vi "Configure External Clock.vi"(0 "device session in":refnum<class "Device Session.lvclass">, 5 "external clock source":T1, 7 "external clock rate (Hz)":dbl=250000000.0 format="%#_6p", 11 "error in":errorcluster) -> (4 "device session out":refnum<class "Device Session.lvclass">, 6 "actual adc clock rate (Hz)":dbl=250000000.0 format="%#_6p", 15 "error out":errorcluster)   [LabVIEW 2021, in "Device Session.lvclass"]
doc: "Selects an external clock source and configures the external clock rate. When using an external clock, you must run the <B>Disable Data Clock</B> VI before disconnecting the external clock source.\n\n<B>Input Parameters</B>\n\n<B>device session in</B> is a reference to the Device Session object, which contains a session to each instrument design library used in this sample project. This parameter is obtained from the 'Open Session' VI.\n\n<B>external clock source</B> specifies the source of the external clock that is divided to become the ADC clock.\n\n'Clock In' (default): specifies that the clock source is the Clock In signal from the device front panel.\n'PXIe DStar A': specifies that the clock source is the signal from the PXIe DStar A line.\n\n<B>external clock rate (Hz)</B> specifies the frequency of the source of the ADC clock. The default value is 250.\n\n<B>error in</B> describes error conditions that occur before this node runs. This input provides standard 'error in' functionality.\n\n<B>Output Parameters</B>\n\n<B>device session out</B> passes a reference to the session to the next VI.\n\n<B>actual adc clock rate (Hz)</B> returns the coerced value of the ADC clock rate.\n\n<B>error out</B> contains error information. This output provides standard 'error out' functionality."
uses:
  Device Session.lvclass
  <instrlib>/HSAI-RIO/Types/v1/Host/Typedefs/External Clock Source.ctl
  Device Session.lvclass/Device Session.ctl
  <instrlib>/HSAI-RIO/Config/Group A/v1/Host/Main/niHSAI Group A Config v1 Host.lvclass
  C:/Program Files (x86)/National Instruments/LabVIEW 2021/instr.lib/HSAI-RIO/Config/Interface/v1/Host/niHSAI Config v1 Host.lvclass
  <instrlib>/HSAI-RIO/Config/Interface/v1/Host/Protected/Configure ADC Clock For External.vi
  <instrlib>/HSAI-RIO/Config/Interface/v1/Host/niHSAI Config v1 Host.lvclass
  C:/Program Files (x86)/National Instruments/LabVIEW 2021/instr.lib/HSAI-RIO/Config/Group A/v1/Host/Main/niHSAI Group A Config v1 Host.lvclass
  <instrlib>/HSAI-RIO/Types/v1/Host/niHSAI Types v1 Host.lvlib
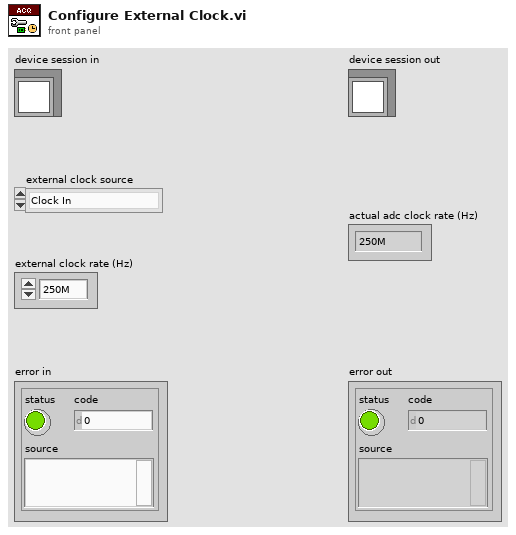
[diagram p1: front panel]
types:
  T1 = typedef "niHSAI Types v1 Host.lvlib/External Clock Source.ctl" = enum8{"Clock In", "PXIe DStar A", "AUX 0 Clock In"}
  T2 = typedef "Device Session.lvclass/Device Session Object.ctl" = cluster{"fpga reference":T3, "reg bus":refnum<class "niInstr FIFO Register Bus v1 Host.lvclass">, "subsystem map":refnum<class "niInstr Subsystem Map v1 Host.lvclass">, "cal data":refnum<class "niHSAI Cal Data v1 Host.lvclass">, "config":refnum<class "niHSAI Group A Config v1 Host.lvclass">, "acquisition 0":refnum<class "niInstr Multirecord Acquisition v1 Host.lvclass">, "acquisition 1":refnum<class "niInstr Multirecord Acquisition v1 Host.lvclass">, "number of selected acq channels":u8, "selected acq channels":bool[], "number of channels":u32, "configured channels":bool[], "acq configuration":cluster{"number of samples":u64, "number of records":u64, "pretrigger samples":u64}, "actual channel configuration":T4[], "sample clock rate (Hz)":dbl, "scaling coefficients":T8[]}
  T3 = typedef "Device Session.lvclass/FPGA Refnum.ctl" = refnum<k20>
  T4 = typedef "niHSAI Types v1 Host.lvlib/Channel Configuration.ctl" = cluster{"channel":u32, "coupling":T5, "impedance":T6, "bandwidth":T7, "vertical range":dbl, "vertical offset":dbl}
  T5 = typedef "niHSAI Types v1 Host.lvlib/Coupling.ctl" = enum8{"Default", "DC", "AC"}
  T6 = typedef "niHSAI Types v1 Host.lvlib/Impedance.ctl" = enum8{"Default", "1 mega ohm", "50 ohm"}
  T7 = typedef "niHSAI Types v1 Host.lvlib/Bandwidth.ctl" = enum8{"Default", "Full Bandwidth", "Anti-alias Filter", "150 MHz"}
  T8 = typedef "niInstr Multirecord Acquisition v1 Host.lvclass/Scaling Coefficient.ctl" = cluster{"gain":dbl, "offset":dbl}
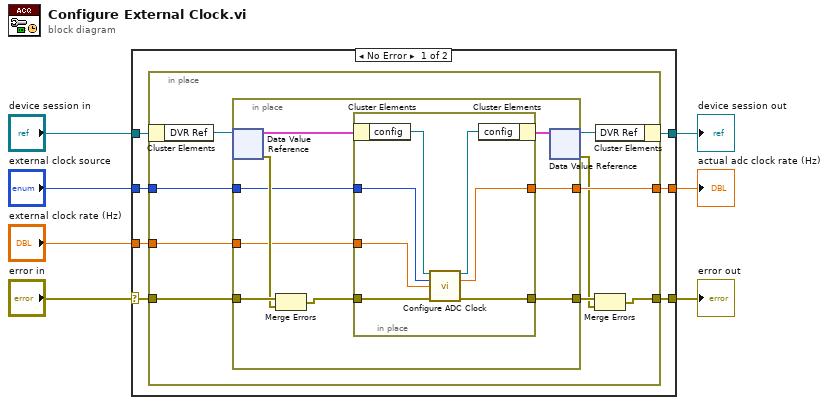
[diagram p0: block diagram]
diagram:
  n1 = case shown="No Error" "error in" {
    selector: "error in" -> [w14 w41]
    tunnel: "device session in" -> [w9 w40]
    tunnel: [w8 w40] -> w1
    tunnel: [w11 w41] -> w3
    tunnel: [w13 _] -> w2
    tunnel: "external clock rate (Hz)" -> [w12 _]
    tunnel: "external clock source" -> [w10 _]
    frame No Error {
      n2 = in-place {
        in-place-border: w14 -> [w23]
        in-place-border: [w22] -> w13
        in-place-border: w12 -> [w20]
        in-place-border: [w15] -> w11
        in-place-border: w10 -> [w18]
        n3 = in-place-cluster #1(w9) -> ("DVR Ref"=w17:refnum<data-value>)
        n4 = in-place {
          in-place-border: w23 -> [w31]
          in-place-border: [w25] -> w22
          in-place-border: [w32] -> w21
          in-place-border: w20 -> [w27]
          in-place-border: w18 -> [w26]
          n5 = in-place-dvr #2(w17) -> (w28:T2, w30:errorcluster)
          n6 = Merge Errors(w31, w30) -> (w29:errorcluster)
          n7 = in-place {
            in-place-border: [w39] -> w32
            in-place-border: w29 -> [w38]
            in-place-border: w27 -> [w37]
            in-place-border: w26 -> [w36]
            in-place-border: [w34] -> w25
            n8 = in-place-cluster #3(w28) -> ("config"=w35:refnum<class "niHSAI Group A Config v1 Host.lvclass">)
            n9 = call-poly <instrlib>:"Configure ADC Clock.vi"("session in"=w35, "external clock source"=w36, "external clock rate (Hz)"=w37, "error in"=w38) -> ("session out"=w33:refnum<class "niHSAI Group A Config v1 Host.lvclass">, "actual adc clock rate (Hz)"=w34:dbl, "error out"=w39:errorcluster)  [unwired: 8 in, 1 out]
            n10 = in-place-cluster #3("config"=w33) -> (w24:T2)
          }
          n11 = in-place-dvr #2(w24) -> (w16:refnum<data-value>, w19:errorcluster)
        }
        n12 = Merge Errors(w21, w19) -> (w15:errorcluster)
        n13 = in-place-cluster #1("DVR Ref"=w16) -> (w8:refnum<class "Device Session.lvclass">)
      }
    }
    frame Error {
    }
  }
  "error out" <- w3
  "device session out" <- w1
  "actual adc clock rate (Hz)" <- w2
